vi "Convert Device Units to Speed Units (FW7).vi"(9 "Microstep Size (0)":dbl, 10 "Units (0: device speed units)":u16(ring) items=["device speed units", "microns per second", "millimeters per second", "inches per second", "degrees per second"], 11 "Device Speed (0)":i64) -> (3 "Speed":dbl)   [LabVIEW 2013, in "Zaber A Series.lvlib"]
doc: "Helper to convert device-specific speed units to standard units of speed.\n\nSelect a unit to convert to and enter a speed measurement from a Zaber device. The measurement will be converted to the selected units.\n\nIf you select a unit other than device speed units, you must also provide the Microstep Size conversion factor from microsteps to micrometers (for linear stages) or degrees (for rotary stages), which can be found in your device manual."
uses:
  Zaber A Series.lvlib
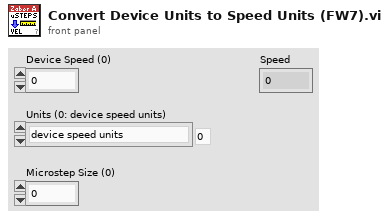
[diagram p1: front panel]
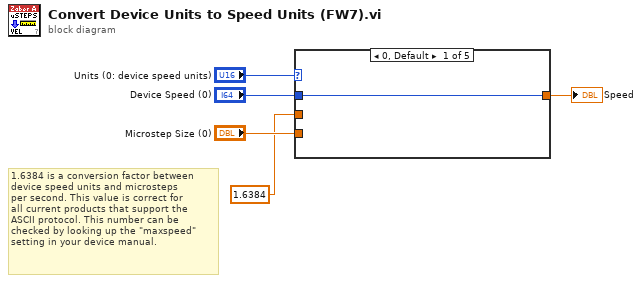
[diagram p0: block diagram]
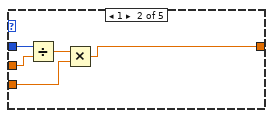
[diagram p2: hidden frame]
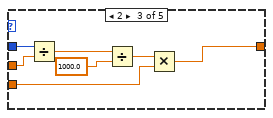
[diagram p3: hidden frame]
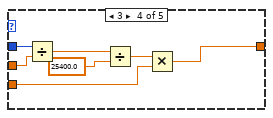
[diagram p4: hidden frame]
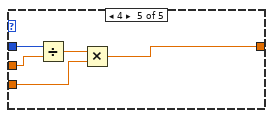
[diagram p5: hidden frame]
diagram:
  # "1.6384 is a conversion factor between \ndevice speed units and microsteps \nper second. This value is correct for\nall current products that support the\nASCII protocol. This number can be \nchecked by looking up the \"maxspeed\"\nsetting in your device manual."
  n1 = case shown="0, Default" "Units (0: device speed units)" {
    tunnel: 1.6384 ("Speed Constant (1.6384)") -> [_ w10 w17 w21 w29]
    tunnel: "Microstep Size (0)" -> [_ w8 w13 w20 w27]
    tunnel: "Device Speed (0)" -> [w6 w11 w18 w22 w30]
    tunnel: [w6 w7 w12 w19 w26] -> w1
    frame 0, Default {
    }
    frame 1 {
      n2 = Divide(x=w11, y=w10) -> (x/y=w9:dbl)
      n3 = Multiply(x=w9, y=w8) -> (x*y=w7:dbl)
    }
    frame 2 {
      n4 = Divide(x=w18, y=w17) -> (x/y=w16:dbl)
      n5 = Divide(x=w16, y=1000.0) -> (x/y=w14:dbl)
      n6 = Multiply(x=w14, y=w13) -> (x*y=w12:dbl)
    }
    frame 3 {
      n7 = Divide(x=w22, y=w21) -> (x/y=w25:dbl)
      n8 = Divide(x=w25, y=25400.0) -> (x/y=w23:dbl)
      n9 = Multiply(x=w23, y=w20) -> (x*y=w19:dbl)
    }
    frame 4 {
      n10 = Divide(x=w30, y=w29) -> (x/y=w28:dbl)
      n11 = Multiply(x=w28, y=w27) -> (x*y=w26:dbl)
    }
  }
  "Speed" <- w1
